vi "FTW-Actor-LocalMessage-Send.vi"(0 "FTW-ActorInstance In":refnum<class "FTW-ActorInstance.lvclass">, 5 "Message Header":string, 7 "Message Body":string, 11 "error in":errorcluster) -> (15 "error out":errorcluster)   [LabVIEW 2013, in "FTW-ActorInstance.lvclass"]
uses:
  FTW-ActorInstance.lvclass
  Package/Base/FTW-Message.lvclass
  FTW-ActorInstance.lvclass/FTW-ActorInstance.ctl
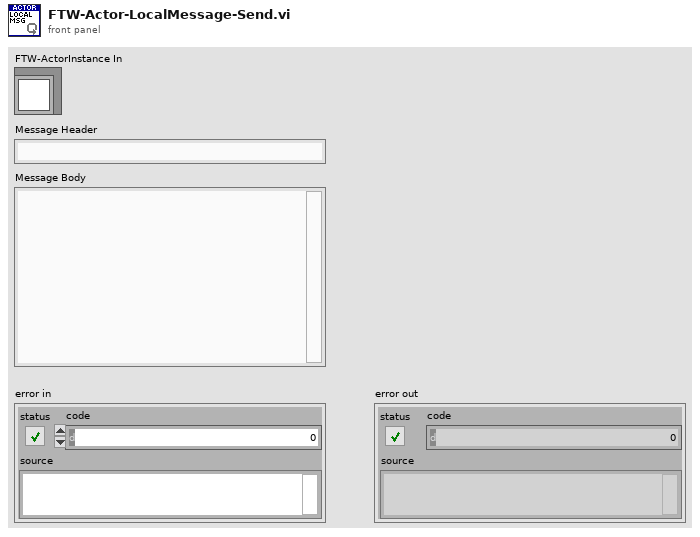
[diagram p1: front panel]
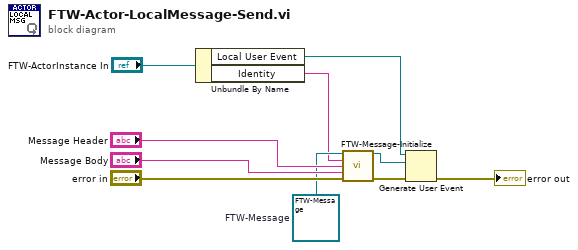
[diagram p0: block diagram]
diagram:
  w3 = refnum<class "FTW-Message.lvclass"> refnum  # FTW-Message
  n1 = Unbundle By Name("FTW-ActorInstance In") -> ("Local User Event"=w2:refnum<user-event>, "Identity"=w1:string)
  n2 = call-dynamic "FTW-Message-Initialize.vi"("FTW Message"=w3, "Sender Identity"=w1, "Message Header"="Message Header", "Message Body"="Message Body", "error in"="error in") -> ("FTW Message out"=w4:refnum<class "FTW-Message.lvclass">, "error out"=w5:errorcluster)  [unwired: 9 in]
  n3 = Generate User Event(user event=w2, event data cluster=w4, error in=w5) -> (error out=→"error out":errorcluster)  [unwired: 1 in, 1 out]
